vi "HelloWorldGUI.vi"() -> ()   [LabVIEW 2014]
panel:
  in  "stop":bool
  in  "Two Tabs":enum32{"First Tab", "Second Tab"}(tab) caption="Tab Control"
  out "Result Message":string
  in  "Message 2":string="Test 2"
  in  "Message 1":string="Test 1"
  in  "Switch Message":bool=TRUE
  in  "Numeric":dbl=5.0
  out "Output":dbl
  in  "Knob":dbl(knob)=9.501356366982368 scale=0.0..40.0
  in  "Method":T1(ring)
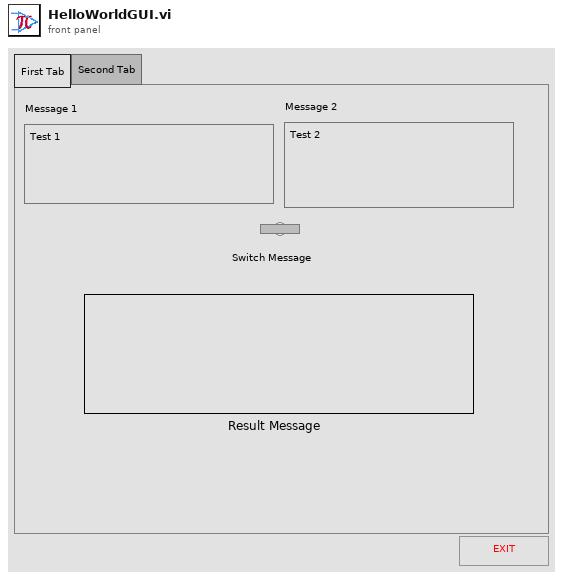
[diagram p1: front panel]
types:
  T1 = enum16{"Reset", "Update From Knob", "Update From Numeric"}
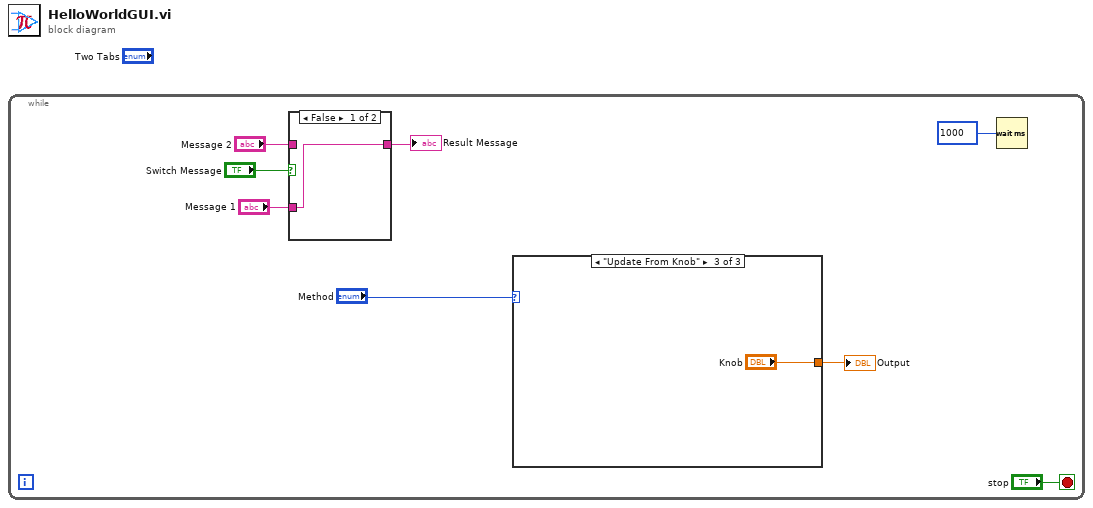
[diagram p0: block diagram]
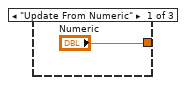
[diagram p3: hidden frame]
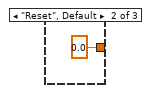
[diagram p4: hidden frame]
diagram:
  n1 = while {
    stop <- "stop" stop-if-true
    n2 = case shown="False" "Switch Message" {
      tunnel: "Message 1" -> [w9 _]
      tunnel: "Message 2" -> [_ w10]
      tunnel: [w9 w10] -> w1
      frame False {
      }
      frame True {
      }
    }
    "Result Message" <- w1
    n3 = case shown="\"Update From Knob\"" "Method" {
      tunnel: ["Numeric" 0.0 ("Knob") "Knob"] -> w5
      frame "Update From Numeric" {
      }
      frame "Reset", Default {
      }
      frame "Update From Knob" {
      }
    }
    "Output" <- w5
    n4 = Wait (ms)(milliseconds to wait=u32 1000) -> ()  [unwired: 1 out]
  }
